vi "Stop Core.vi"(10 "final error code":i32, 11 "EventRecorder In":refnum<class "EventRecorder.lvclass">) -> (3 "EventRecorder Out":refnum<class "EventRecorder.lvclass">)   [LabVIEW 2019, in "EventRecorder.lvlib" / "EventRecorder.lvclass"]
uses:
  EventRecorder.lvclass
  EventRecorder.lvclass/EventRecorder.ctl
  <vilib>/NI/Event Source Actor/Event Source/Event Source/Event Source.lvclass
  <vilib>/NI/Event Logger Library/EventLog/EventLog.lvclass
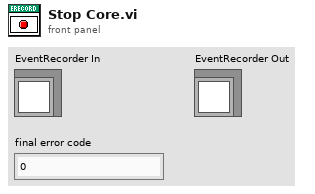
[diagram p1: front panel]
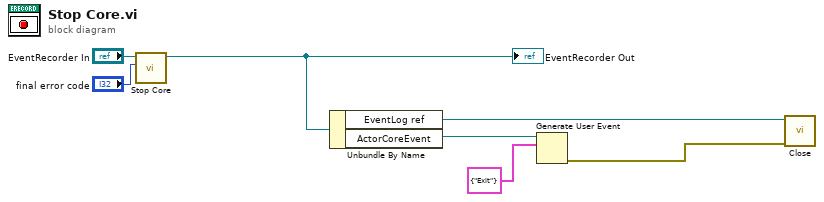
[diagram p0: block diagram]
diagram:
  n1 = call-parent "Stop Core.vi"("final error code"="final error code", "Event Source In"="EventRecorder In") -> ("Event Source Out"=w5:refnum<class "EventRecorder.lvclass">)  [unwired: 9 in]
  "EventRecorder Out" <- w5
  n2 = Unbundle By Name(w5) -> ("EventLog ref"=w4:refnum<class "EventLog.lvclass">, "ActorCoreEvent"=w3:refnum<user-event>)
  n3 = Generate User Event(user event=w3, event data cluster=cluster{"ActorCoreMessage":string} {"ActorCoreMessage"="Exit"} ("event data")) -> (error out=w2:errorcluster)  [unwired: 2 in, 1 out]
  n4 = call <vilib>:"Close.vi"("error in (no error)"=w2, "EventLog ref"=w4) -> ()  [unwired: 9 in, 1 out]
